vi "Look In Registry.vi"(8 "error in (no error)":errorcluster, 10 "Tag Name":string, 11 "Current Value Table in":refnum<class "Current Value Table.lvclass">) -> (0 "error out":errorcluster, 1 "key not found?":bool, 2 "CVT_Item out":refnum<class "iCVT_Item.lvclass">, 3 "Current Value Table out":refnum<class "Current Value Table.lvclass">)   [LabVIEW 2024, in "Current Value Table.lvlib" / "Current Value Table.lvclass"]
uses:
  Current Value Table.lvclass
  iCVT_Item/iCVT_Item.lvclass
  Current Value Table.lvclass/Current Value Table.ctl
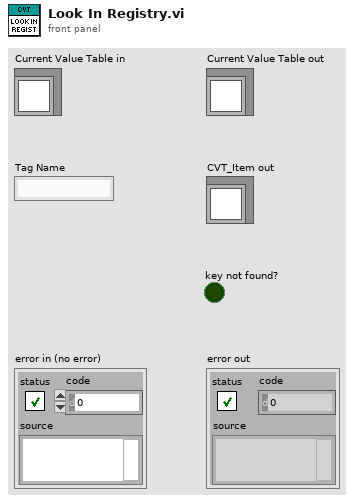
[diagram p1: front panel]
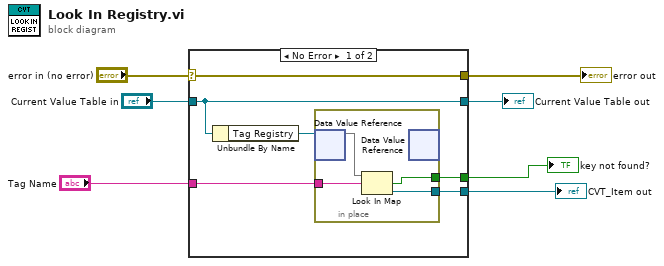
[diagram p0: block diagram]
diagram:
  n1 = case shown="No Error" "error in (no error)" {
    selector: "error in (no error)" -> [w13 w19]
    tunnel: [w13 w19] -> w6
    tunnel: [w12 w18] -> w4
    tunnel: "Current Value Table in" -> [w12 w18]
    tunnel: "Tag Name" -> [w10 _]
    tunnel: [w9 _] -> w2
    tunnel: [w8 _] -> w1
    frame No Error {
      n2 = Unbundle By Name(w12) -> ("Tag Registry"=w11:refnum<data-value>)
      n3 = in-place {
        in-place-border: w10 -> [w16]
        in-place-border: [w15] -> w9
        in-place-border: [w14] -> w8
        n4 = in-place-dvr #1(w11) -> (w17:map{string, refnum<class "iCVT_Item.lvclass">})  [unwired: 1 out]
        n5 = Look In Map(map=w17, key=w16) -> (key not found?=w14:bool, value=w15:refnum<class "iCVT_Item.lvclass">)  [unwired: 1 in]
        n6 = in-place-dvr #1() -> ()  [unwired: 1 in, 2 out]
      }
    }
    frame Error {
    }
  }
  "error out" <- w6
  "Current Value Table out" <- w4
  "CVT_Item out" <- w2
  "key not found?" <- w1
